vi "调整图片亮度.vi"() -> ()   [LabVIEW 2012, in "Picture Box Tools.lvlib"]
uses:
  Picture Box Tools.lvlib
panel:
  in  "L":dbl(slide) scale=0.0..240.0
  in  "S":dbl(slide) scale=0.0..240.0
  in  "H":dbl(slide) scale=0.0..240.0
  out "二维图片":picture
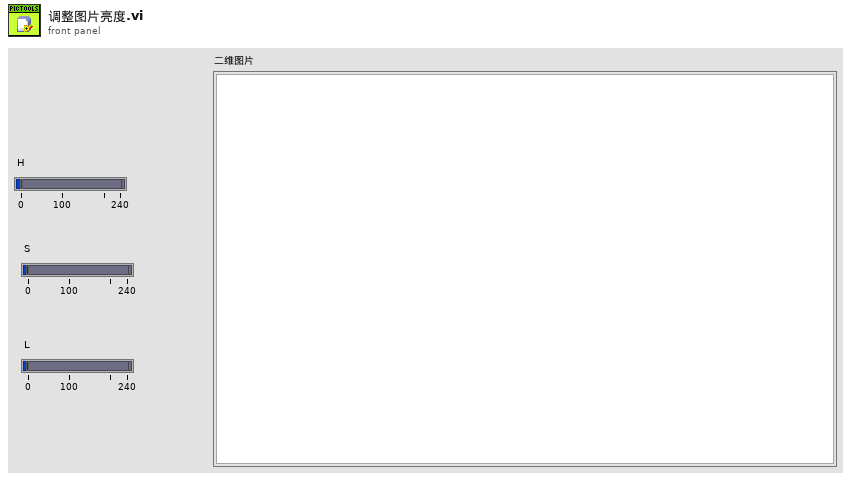
[diagram p1: front panel]
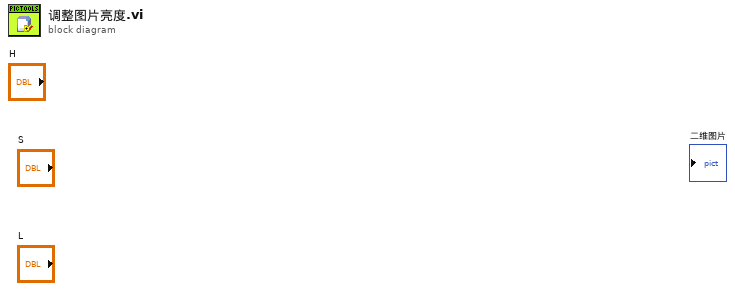
[diagram p0: block diagram]
diagram:
